vi "REWORK_set_IP_and_port_after_connection_established.vi"(8 "error_in":errorcluster, 10 "PLC_port":u16, 11 "PLC_IP":string) -> (0 "error_out":errorcluster)   [LabVIEW 2019]
uses:
  FGV/DIAGNOSTICS_records_display/FGV_REWORK_DIAGNOSTICS_records_display.ctl
  _misc/PLC_connection_status.ctl
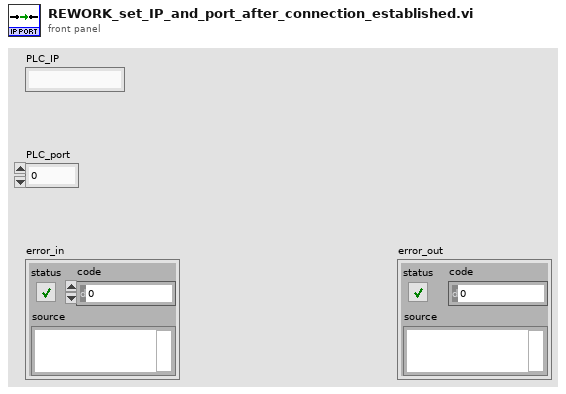
[diagram p1: front panel]
types:
  T1 = typedef "PLC_connection_status.ctl" = enum16{"Connected", "Waiting", "Error", "-"}
  T2 = typedef "FGV_REWORK_DIAGNOSTICS_records_display.ctl" = enum16{"initialize", "set_PLC_IP", "set_PLC_Port", "set_PLC_connection_status", "set_SQL_connection_status", "get_all_info"}
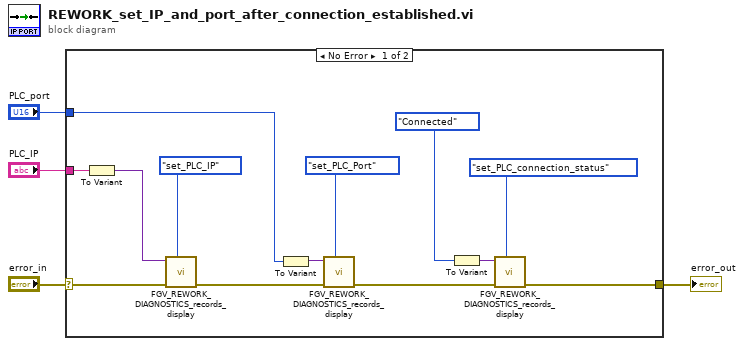
[diagram p0: block diagram]
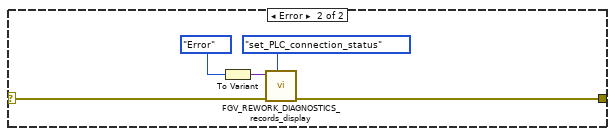
[diagram p2: hidden frame]
diagram:
  n1 = case shown="No Error" "error_in" {
    selector: "error_in" -> [w8 w19]
    tunnel: "PLC_port" -> [w14 _]
    tunnel: "PLC_IP" -> [w11 _]
    tunnel: [w5 w18] -> w1
    frame No Error {
      n2 = To Variant(anything=w11) -> (Variant=w10:variant)
      n3 = call "FGV_REWORK_DIAGNOSTICS_records_display.vi"("options"=FGV_REWORK_DIAGNOSTICS_records_display."set_PLC_IP", "error_in"=w8, "input"=w10) -> ("error_out"=w7:errorcluster)  [unwired: 7 in, 1 out]
      n4 = To Variant(anything=w14) -> (Variant=w13:variant)
      n5 = call "FGV_REWORK_DIAGNOSTICS_records_display.vi"("options"=FGV_REWORK_DIAGNOSTICS_records_display."set_PLC_Port", "error_in"=w7, "input"=w13) -> ("error_out"=w6:errorcluster)  [unwired: 7 in, 1 out]
      n6 = To Variant(anything=PLC_connection_status."Connected" ("connection_status")) -> (Variant=w15:variant)
      n7 = call "FGV_REWORK_DIAGNOSTICS_records_display.vi"("options"=FGV_REWORK_DIAGNOSTICS_records_display."set_PLC_connection_status", "error_in"=w6, "input"=w15) -> ("error_out"=w5:errorcluster)  [unwired: 7 in, 1 out]
    }
    frame Error {
      n8 = To Variant(anything=PLC_connection_status."Error" ("connection_status")) -> (Variant=w20:variant)
      n9 = call "FGV_REWORK_DIAGNOSTICS_records_display.vi"("options"=FGV_REWORK_DIAGNOSTICS_records_display."set_PLC_connection_status", "error_in"=w19, "input"=w20) -> ("error_out"=w18:errorcluster)  [unwired: 7 in, 1 out]
    }
  }
  "error_out" <- w1
